vi "Save Front panel to Image.vi"(8 "error in (no error)":errorcluster, 10 "FileName":string, 11 "CallActorCenter in":refnum<class "CallActorCenter.lvclass">) -> (0 "error out":errorcluster, 3 "CallActorCenter out":refnum<class "CallActorCenter.lvclass">)   [LabVIEW 2021, in "CallActorCenter.lvclass"]
uses:
  CallActorCenter.lvclass
  CallActorCenter.lvclass/CallActorCenter.ctl
  <vilib>/ActorFramework/Actor/Actor.lvclass
  <userlib>/John_Lib/Interfaces/FrontPanel Save Image Messages/Save Front panel to Image Msg/Save Front panel to Image Msg.lvclass
  C:/Program Files (x86)/National Instruments/LabVIEW 2021/user.lib/John_Lib/AbstractActorTemplate/AbstractActorTemplate/UIActorTop.lvclass
  C:/Program Files (x86)/National Instruments/LabVIEW 2021/vi.lib/ActorFramework/Actor/Actor.lvclass
  C:/Program Files (x86)/National Instruments/LabVIEW 2021/project/Create Actor from Template/_CallActorCenter/CallActorCenter.lvclass
  C:/Program Files (x86)/National Instruments/LabVIEW 2021/user.lib/John_Lib/Interfaces/InsertLeftSubPanel/InsertLeftSubPanel.lvclass
  C:/Program Files (x86)/National Instruments/LabVIEW 2021/user.lib/John_Lib/Interfaces/InsertMainSubPanel/InsertMainSubPanel.lvclass
  C:/Program Files (x86)/National Instruments/LabVIEW 2021/user.lib/John_Lib/Interfaces/InsertRightSubPanel/InsertRightSubPanel.lvclass
  C:/Program Files (x86)/National Instruments/LabVIEW 2021/user.lib/John_Lib/Interfaces/FrontPanel Save Image/FrontPanel Save Image.lvclass
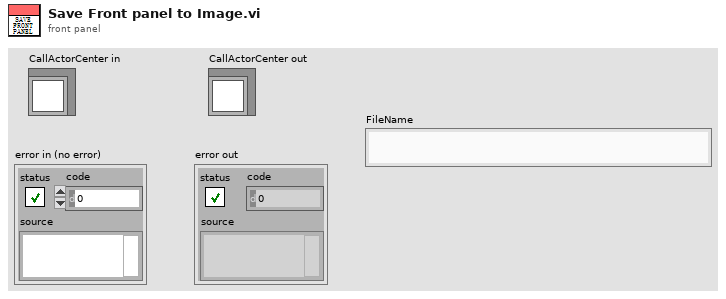
[diagram p1: front panel]
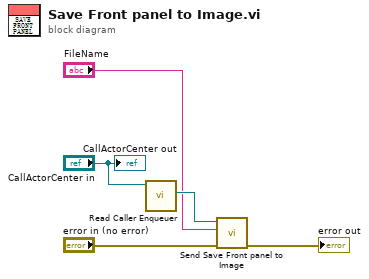
[diagram p0: block diagram]
diagram:
  n1 = call <vilib>:"Read Caller Enqueuer.vi"("Actor"="CallActorCenter in") -> ("Caller Enqueuer"=w4:refnum<class "Message Enqueuer.lvclass">)  [unwired: 10 in]
  n2 = call <userlib>:"Send Save Front panel to Image.vi"("error in (no error)"="error in (no error)", "FileName"="FileName", "Message Enqueuer"=w4) -> ("error out"=→"error out":errorcluster)  [unwired: 7 in, 1 out]
  "CallActorCenter out" <- "CallActorCenter in"
